vi "RDG822 User(before_screen_branch).vi"() -> ()   [LabVIEW 2021]
panel:
  in  "RemoveReq?":bool
  in  "userID":string="0001"
  out "error out":errorcluster
  in  "E:\\Study\\НИР_Маг\\FP":path=path "E:/Study/НИР_Маг/FP"
  in  "error in":errorcluster
  in  "PhaseDBL":dbl format="%.3f"
  in  "OK":bool
  out "Screen\nPhase":picture
  out "PhaseStr":string="5.0000"
  in  "LowL":dbl=-2.5 format="%.4f"
  in  "Offset":dbl format="%.4f"
  out "Screen\nOffset-LowL":picture
  out "Offset-LowL":string="5.0000"
  in  "Offset/LowL":bool
  in  "HighL":dbl=1.0 format="%.4f"
  in  "Ampl":dbl=5.0 format="%.4f"
  out "Screen\nAmpl-HighL":picture
  out "Ampl-HighL":string="5.0000"
  in  "Ampl/HighL":bool
  in  "Freq":dbl=1.0 format="%.18f"
  in  "Period":dbl=1.0 format="%_8g"
  out "Screen\nFreq/Period":picture
  out "Freq-Period":string="1,000000000"
  in  "Freq/Period":bool
  in  "Left":bool
  in  "Right":bool
  in  "Out2":bool
  in  "Out1":bool
  out "Screen":picture
  in  "Menu":bool
  in  "Home":bool
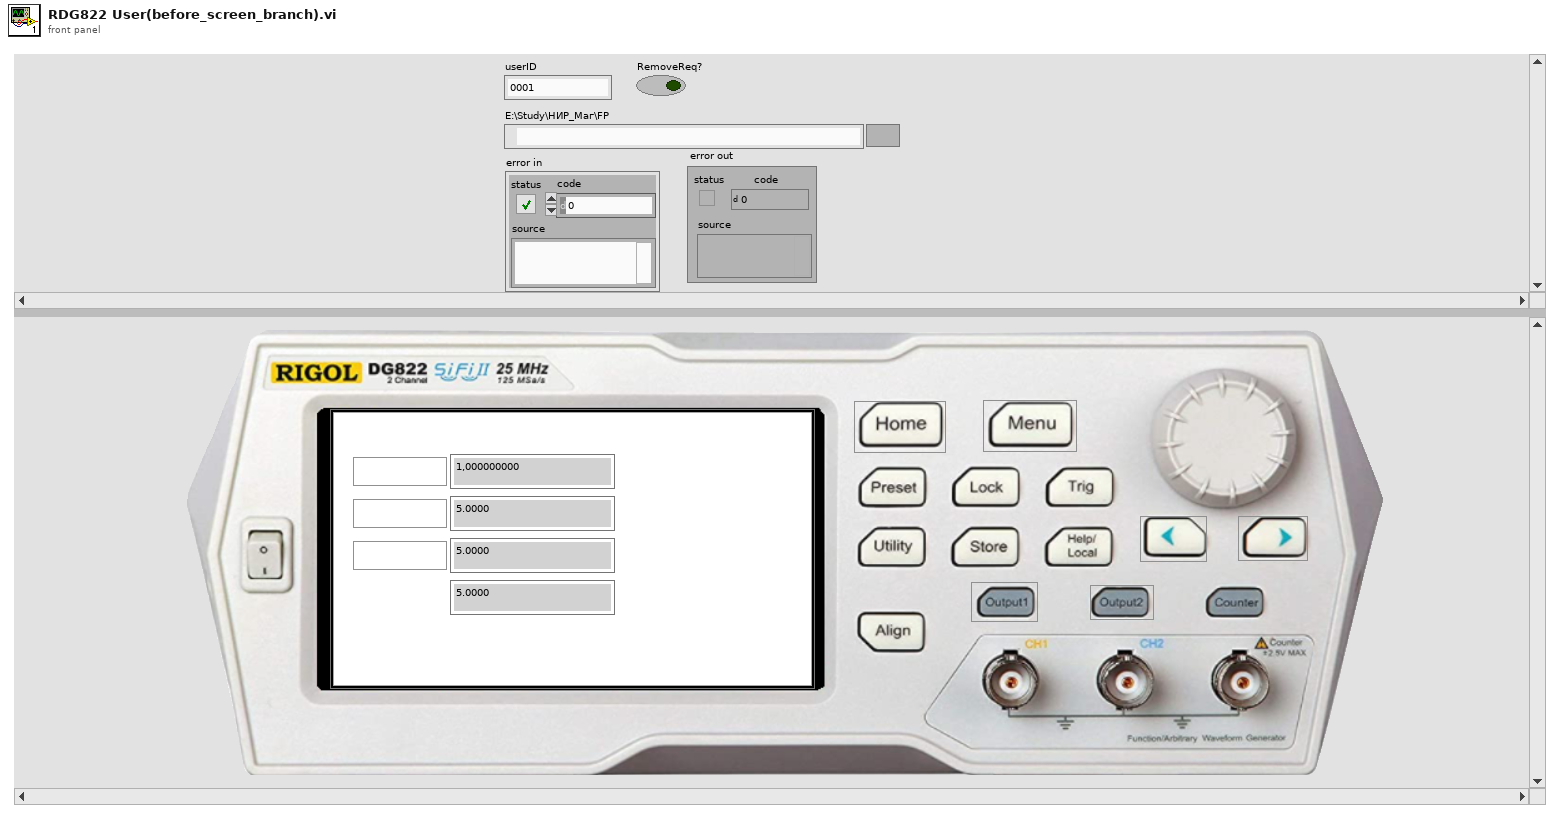
[diagram p1: front panel]
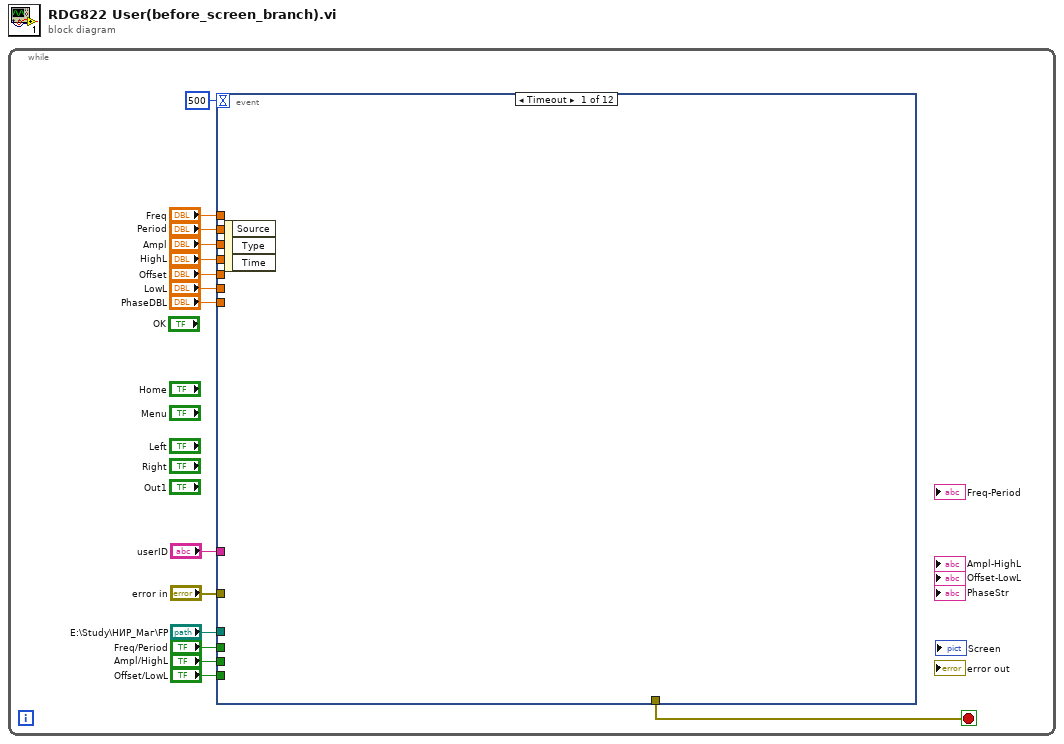
[diagram p0: block diagram]
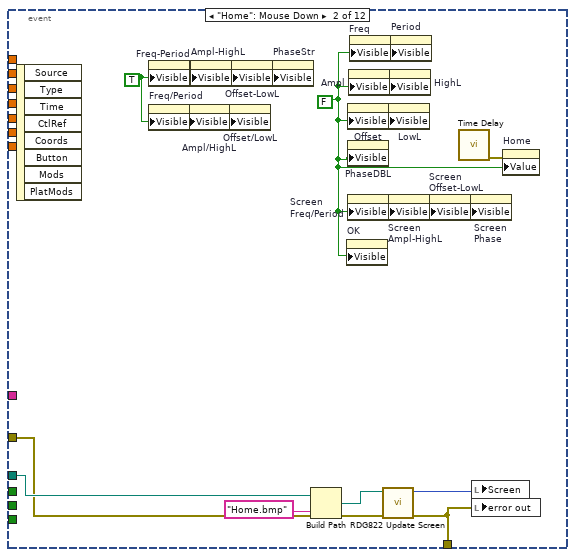
[diagram p2: hidden frame]
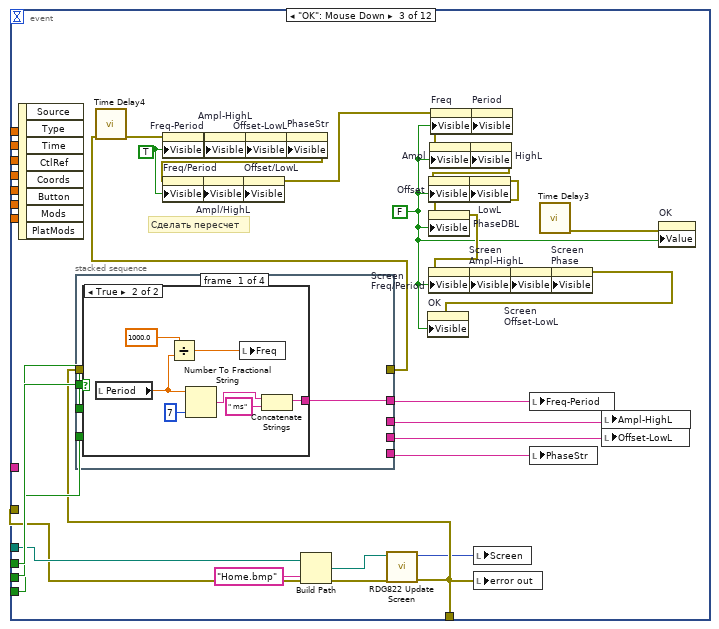
[diagram p3: hidden frame]
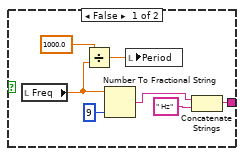
[diagram p4: hidden frame]
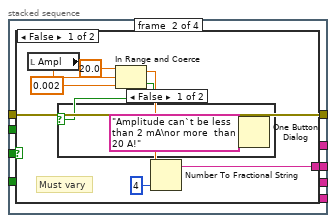
[diagram p5: hidden frame]
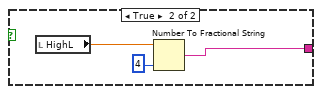
[diagram p7: hidden frame]
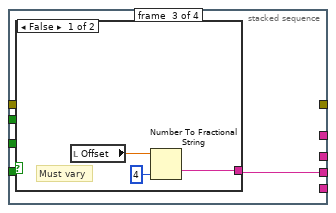
[diagram p8: hidden frame]
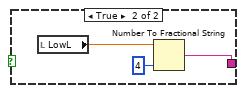
[diagram p9: hidden frame]
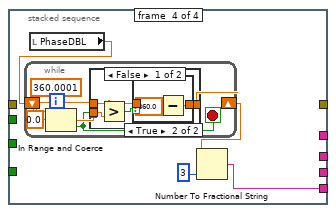
[diagram p10: hidden frame]
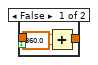
[diagram p11: hidden frame]
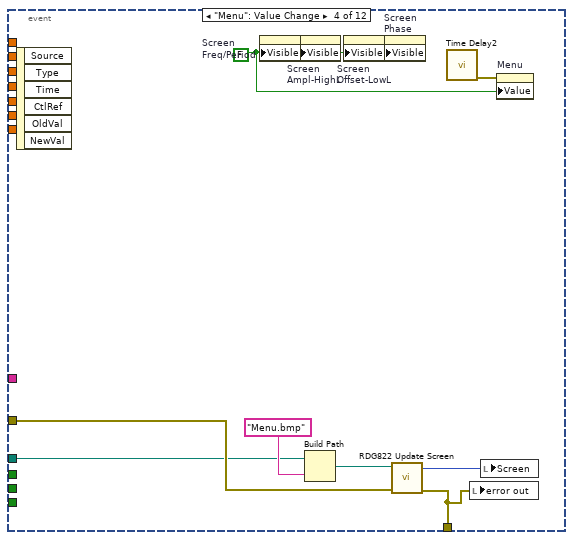
[diagram p13: hidden frame]
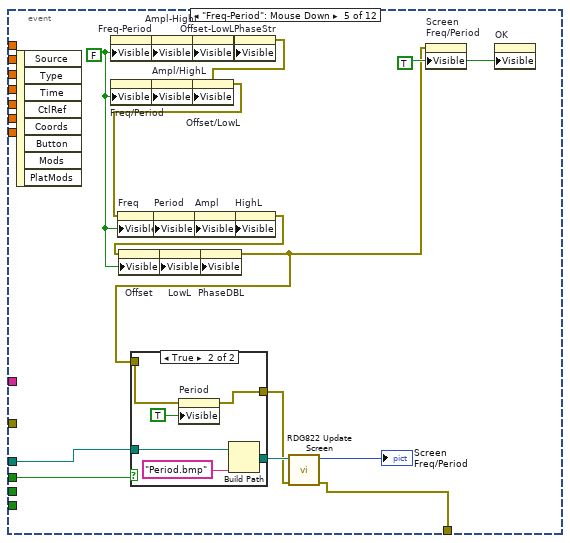
[diagram p14: hidden frame]
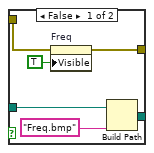
[diagram p15: hidden frame]
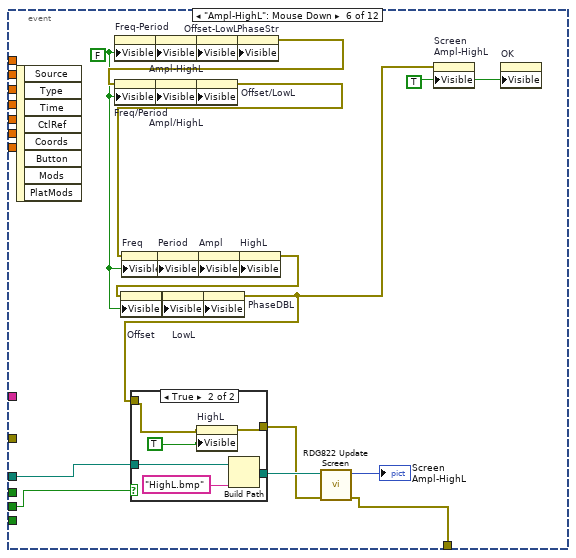
[diagram p16: hidden frame]
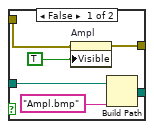
[diagram p17: hidden frame]
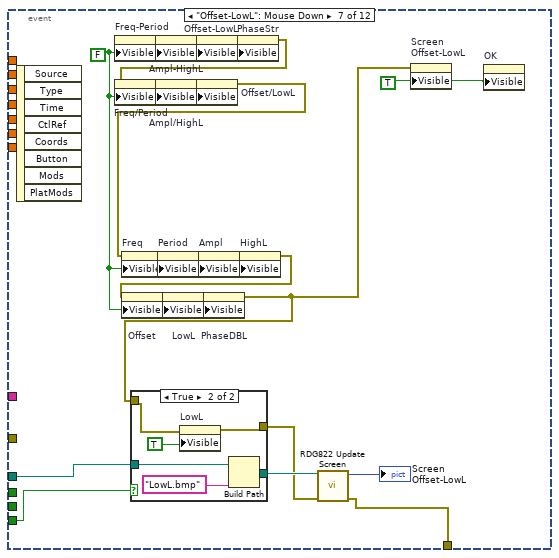
[diagram p18: hidden frame]
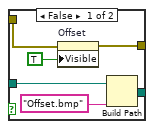
[diagram p19: hidden frame]
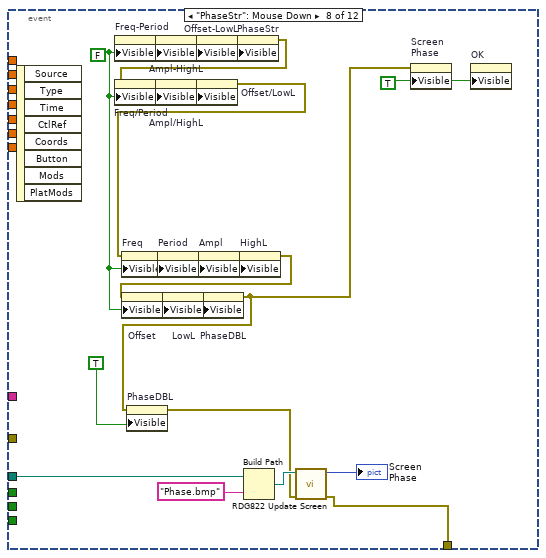
[diagram p20: hidden frame]
diagram:
  n1 = while {
    stop <- w15 stop-if-true
    n2 = event shown="[0] Timeout" {
      selector: _ -> [_ _ _ _ _ _ _ _ _ _ _ _]
      dyn-events: _ -> [_ _ _ _ _ _ _ _ _ _ _ _]
      timeout: 500 -> [_ _ _ _ _ _ _ _ _ _ _ _]
      tunnel: [_ w19 w28 w120 w127 w161 w195 w229 _ _ w296 w374] -> w15
      tunnel: "error in" -> [_ w18 w27 w122 _ _ _ _ _ _ w306 _]
      tunnel: "E:\\Study\\НИР_Маг\\FP" -> [_ w20 w29 w121 w148 w182 w216 w238 _ _ w288 w373]
      tunnel: "Freq/Period" -> [_ _ w35 _ w146 _ _ _ _ _ w325 _]
      tunnel: "Ampl/HighL" -> [_ _ w34 _ _ w177 _ _ _ _ w326 _]
      tunnel: "Freq" -> [_ _ _ _ _ _ _ _ _ _ w324 _]
      tunnel: "Ampl" -> [_ _ _ _ _ _ _ _ _ _ w322 _]
      tunnel: "Period" -> [_ _ _ _ _ _ _ _ _ _ w323 _]
      tunnel: "HighL" -> [_ _ _ _ _ _ _ _ _ _ w318 _]
      tunnel: "Offset/LowL" -> [_ _ w33 _ _ _ w203 _ _ _ w321 _]
      tunnel: "Offset" -> [_ _ _ _ _ _ _ _ _ _ w320 _]
      tunnel: "LowL" -> [_ _ _ _ _ _ _ _ _ _ w319 _]
      tunnel: "PhaseDBL" -> [_ _ _ _ _ _ _ _ _ _ w312 _]
      tunnel: "userID" -> [_ _ _ _ _ _ _ _ _ _ w301 _]
      event Timeout {
        n3 = event-data() -> ()  [unwired: 1 in, 3 out]
      }
      event "Home": Mouse Down {
        w23 = TRUE ("Visible")
        w22 = FALSE ("Visible")
        n4 = event-data() -> ()  [unwired: 1 in, 8 out]
        n5 = property on="Freq-Period" class="Str"("Visible"=w23) -> ()  [unwired: 2 in, 2 out]
        n6 = property on="Freq/Period" class="Bool (strict)"("Visible"=w23) -> ()  [unwired: 2 in, 2 out]
        n7 = property on="Ampl/HighL" class="Bool (strict)"("Visible"=w23) -> ()  [unwired: 2 in, 2 out]
        n8 = property on="Ampl-HighL" class="Str"("Visible"=w23) -> ()  [unwired: 2 in, 2 out]
        n9 = property on="Offset/LowL" class="Bool (strict)"("Visible"=w23) -> ()  [unwired: 2 in, 2 out]
        n10 = property on="Offset-LowL" class="Str"("Visible"=w23) -> ()  [unwired: 2 in, 2 out]
        n11 = property on="PhaseStr" class="Str"("Visible"=w23) -> ()  [unwired: 2 in, 2 out]
        n12 = Build Path(base path=w20, name or relative path="Home.bmp") -> (appended path=w17:path)
        n13 = property on="OK" class="Bool (strict)"("Visible"=w22) -> ()  [unwired: 2 in, 2 out]
        n14 = property on="Offset" class="DigNum (strict)"("Visible"=w22) -> ()  [unwired: 2 in, 2 out]
        n15 = property on="PhaseDBL" class="DigNum (strict)"("Visible"=w22) -> ()  [unwired: 2 in, 2 out]
        n16 = property on="Screen\nFreq/Period" class="Pict"("Visible"=w22) -> ()  [unwired: 2 in, 2 out]
        n17 = property on="Ampl" class="DigNum (strict)"("Visible"=w22) -> ()  [unwired: 2 in, 2 out]
        n18 = property on="Freq" class="DigNum (strict)"("Visible"=w22) -> ()  [unwired: 2 in, 2 out]
        n19 = call "RDG822 Update Screen.vi"("error in"=w18, "Path to file"=w17) -> ("error out"=w19:errorcluster, "Screen"=w16:picture)  [unwired: 8 in]
        n20 = property on="LowL" class="DigNum (strict)"("Visible"=w22) -> ()  [unwired: 2 in, 2 out]
        n21 = property on="Screen\nAmpl-HighL" class="Pict"("Visible"=w22) -> ()  [unwired: 2 in, 2 out]
        n22 = property on="HighL" class="DigNum (strict)"("Visible"=w22) -> ()  [unwired: 2 in, 2 out]
        n23 = property on="Period" class="DigNum (strict)"("Visible"=w22) -> ()  [unwired: 2 in, 2 out]
        n24 = property on="Screen\nOffset-LowL" class="Pict"("Visible"=w22) -> ()  [unwired: 2 in, 2 out]
        n25 = call "Time Delay"() -> ("error out"=w24:errorcluster)  [unwired: 11 in]
        n26 = property on="Screen\nPhase" class="Pict"("Visible"=w22) -> ()  [unwired: 2 in, 2 out]
        n27 = local write "Screen"(w16) -> ()
        n28 = local write "error out"(w19) -> ()
        n29 = property on="Home" class="Bool (strict)"(error in=w24, "Value"=w22) -> ()  [unwired: 1 in, 2 out]
      }
      event "OK": Mouse Down {
        w59 = TRUE ("Visible")
        w39 = FALSE ("Visible")
        # "Сделать пересчет"
        n30 = event-data() -> ()  [unwired: 1 in, 8 out]
        n31 = Build Path(base path=w29, name or relative path="Home.bmp") -> (appended path=w26:path)
        n32 = call "RDG822 Update Screen.vi"("error in"=w27, "Path to file"=w26) -> ("error out"=w28:errorcluster, "Screen"=w25:picture)  [unwired: 8 in]
        n33 = stacked-sequence {
          tunnel: [_ _ w92 _] -> w38
          tunnel: [_ w79 _ _] -> w37
          tunnel: [w62 _ _ _] -> w36
          tunnel: w35 -> [w61 _ _ _]
          tunnel: w34 -> [_ w78 _ _]
          tunnel: w33 -> [_ _ w91 _]
          tunnel: [_ w77 _ _] -> w32
          tunnel: w28 -> [_ w77 _ _]
          tunnel: [_ _ _ w101] -> w31
          frame #0 {
            n34 = case shown="True" w61 {
              tunnel: [w64 w71] -> w62
              frame False {
                n35 = local read "Freq"() -> (w67:dbl)
                n36 = Divide(x=1000.0, y=w67) -> (x/y=w66:dbl)
                n37 = Number To Fractional String(number=w67, precision (6)=i16 9) -> (F-format string=w63:string)  [unwired: 2 in]
                n38 = local write "Period"(w66) -> ()
                n39 = Concatenate Strings(w63, " Hz" ("string")) -> (w64:string)
              }
              frame True {
                n40 = local read "Period"() -> (w74:dbl)
                n41 = Divide(x=1000.0, y=w74) -> (x/y=w73:dbl)
                n42 = Number To Fractional String(number=w74, precision (6)=i16 7) -> (F-format string=w70:string)  [unwired: 2 in]
                n43 = local write "Freq"(w73) -> ()
                n44 = Concatenate Strings(w70, " ms" ("string")) -> (w71:string)
              }
            }
          }
          frame #1 {
            n45 = case shown="False" w78 {
              tunnel: [w85 w88] -> w79
              frame False {
                # "Must vary"
                n46 = local read "Ampl"() -> (w84:dbl)
                n47 = In Range and Coerce(upper limit=20.0, x=w84, lower limit=0.002 ("t")) -> (coerced(x)=w81:dbl, In Range?=w80:bool)
                n48 = case shown="False" w80 {
                  frame False {
                    n49 = One Button Dialog(message="Amplitude can`t be less than 2 mA\nor more  than 20 A!") -> ()  [unwired: 1 in, 1 out]
                  }
                  frame True {
                  }
                }
                n50 = Number To Fractional String(number=w81, precision (6)=i16 4) -> (F-format string=w85:string)  [unwired: 2 in]
              }
              frame True {
                n51 = local read "HighL"() -> (w89:dbl)
                n52 = Number To Fractional String(number=w89, precision (6)=i16 4) -> (F-format string=w88:string)  [unwired: 2 in]
              }
            }
          }
          frame #2 {
            n53 = case shown="False" w91 {
              tunnel: [w94 w98] -> w92
              frame False {
                # "Must vary"
                n54 = local read "Offset"() -> (w95:dbl)
                n55 = Number To Fractional String(number=w95, precision (6)=i16 4) -> (F-format string=w94:string)  [unwired: 2 in]
              }
              frame True {
                n56 = local read "LowL"() -> (w96:dbl)
                n57 = Number To Fractional String(number=w96, precision (6)=i16 4) -> (F-format string=w98:string)  [unwired: 2 in]
              }
            }
          }
          frame #3 {
            n58 = local read "PhaseDBL"() -> (w100:dbl)
            n59 = while {
              shift-right: [w103] -> w99
              shift-left: w100 -> [w105]
              stop <- w104 stop-if-true
              w106 = 360.0001 ("upper limit")
              n60 = In Range and Coerce(upper limit=w106, x=w105, lower limit=0.0) -> (In Range?=w104:bool)  [unwired: 1 out]
              n61 = case shown="False" w104 {
                tunnel: w106 -> [w111 _]
                tunnel: w105 -> [w109 w118]
                tunnel: [w108 w118] -> w103
                frame False {
                  n62 = Greater?(x=w109, y=w111) -> (0:w110:bool)
                  n63 = case shown="True" w110 {
                    tunnel: w109 -> [w113 w115]
                    tunnel: [w112 w116] -> w108
                    frame False {
                      n64 = Add(x=w113, y=360.0) -> (x+y=w112:dbl)
                    }
                    frame True {
                      n65 = Subtract(x=w115, y=360.0) -> (x-y=w116:dbl)
                    }
                  }
                }
                frame True {
                }
              }
            }
            n66 = Number To Fractional String(number=w99, precision (6)=i16 3) -> (F-format string=w101:string)  [unwired: 2 in]
          }
        }
        n67 = call "Time Delay4"("error in (no error)"=w32) -> ("error out"=w58:errorcluster)  [unwired: 10 in]
        n68 = property on="Freq-Period" class="Str"(error in=w58, "Visible"=w59) -> (error out=w57:errorcluster)  [unwired: 1 in, 1 out]
        n69 = property on="Ampl-HighL" class="Str"(error in=w57, "Visible"=w59) -> (error out=w56:errorcluster)  [unwired: 1 in, 1 out]
        n70 = property on="Offset-LowL" class="Str"(error in=w56, "Visible"=w59) -> (error out=w55:errorcluster)  [unwired: 1 in, 1 out]
        n71 = property on="PhaseStr" class="Str"(error in=w55, "Visible"=w59) -> (error out=w54:errorcluster)  [unwired: 1 in, 1 out]
        n72 = property on="Freq/Period" class="Bool (strict)"(error in=w54, "Visible"=w59) -> (error out=w53:errorcluster)  [unwired: 1 in, 1 out]
        n73 = property on="Ampl/HighL" class="Bool (strict)"(error in=w53, "Visible"=w59) -> (error out=w52:errorcluster)  [unwired: 1 in, 1 out]
        n74 = property on="Offset/LowL" class="Bool (strict)"(error in=w52, "Visible"=w59) -> (error out=w51:errorcluster)  [unwired: 1 in, 1 out]
        n75 = property on="Freq" class="DigNum (strict)"(error in=w51, "Visible"=w39) -> (error out=w50:errorcluster)  [unwired: 1 in, 1 out]
        n76 = property on="Period" class="DigNum (strict)"(error in=w50, "Visible"=w39) -> (error out=w49:errorcluster)  [unwired: 1 in, 1 out]
        n77 = property on="Ampl" class="DigNum (strict)"(error in=w49, "Visible"=w39) -> (error out=w48:errorcluster)  [unwired: 1 in, 1 out]
        n78 = property on="HighL" class="DigNum (strict)"(error in=w48, "Visible"=w39) -> (error out=w47:errorcluster)  [unwired: 1 in, 1 out]
        n79 = property on="Offset" class="DigNum (strict)"(error in=w47, "Visible"=w39) -> (error out=w46:errorcluster)  [unwired: 1 in, 1 out]
        n80 = property on="LowL" class="DigNum (strict)"(error in=w46, "Visible"=w39) -> (error out=w41:errorcluster)  [unwired: 1 in, 1 out]
        n81 = property on="PhaseDBL" class="DigNum (strict)"(error in=w41, "Visible"=w39) -> (error out=w40:errorcluster)  [unwired: 1 in, 1 out]
        n82 = property on="Screen\nFreq/Period" class="Pict"(error in=w40, "Visible"=w39) -> (error out=w45:errorcluster)  [unwired: 1 in, 1 out]
        n83 = property on="Screen\nAmpl-HighL" class="Pict"(error in=w45, "Visible"=w39) -> (error out=w44:errorcluster)  [unwired: 1 in, 1 out]
        n84 = local write "Screen"(w25) -> ()
        n85 = local write "error out"(w28) -> ()
        n86 = property on="Screen\nOffset-LowL" class="Pict"(error in=w44, "Visible"=w39) -> (error out=w43:errorcluster)  [unwired: 1 in, 1 out]
        n87 = local write "Freq-Period"(w36) -> ()
        n88 = local write "PhaseStr"(w31) -> ()
        n89 = call "Time Delay3"() -> ("error out"=w60:errorcluster)  [unwired: 11 in]
        n90 = property on="Screen\nPhase" class="Pict"(error in=w43, "Visible"=w39) -> (error out=w42:errorcluster)  [unwired: 1 in, 1 out]
        n91 = property on="OK" class="Bool (strict)"(error in=w42, "Visible"=w39) -> ()  [unwired: 1 in, 2 out]
        n92 = local write "Ampl-HighL"(w37) -> ()
        n93 = local write "Offset-LowL"(w38) -> ()
        n94 = property on="OK" class="Bool (strict)"(error in=w60, "Value"=w39) -> ()  [unwired: 1 in, 2 out]
      }
      event "Menu": Value Change {
        w125 = FALSE ("Visible")
        n95 = event-data() -> ()  [unwired: 1 in, 6 out]
        n96 = property on="Screen\nFreq/Period" class="Pict"("Visible"=w125) -> ()  [unwired: 2 in, 2 out]
        n97 = property on="Screen\nAmpl-HighL" class="Pict"("Visible"=w125) -> ()  [unwired: 2 in, 2 out]
        n98 = Build Path(base path=w121, name or relative path="Menu.bmp") -> (appended path=w123:path)
        n99 = property on="Screen\nOffset-LowL" class="Pict"("Visible"=w125) -> ()  [unwired: 2 in, 2 out]
        n100 = property on="Screen\nPhase" class="Pict"("Visible"=w125) -> ()  [unwired: 2 in, 2 out]
        n101 = call "RDG822 Update Screen.vi"("error in"=w122, "Path to file"=w123) -> ("error out"=w120:errorcluster, "Screen"=w119:picture)  [unwired: 8 in]
        n102 = call "Time Delay2"() -> ("error out"=w126:errorcluster)  [unwired: 11 in]
        n103 = local write "error out"(w120) -> ()
        n104 = local write "Screen"(w119) -> ()
        n105 = property on="Menu" class="Bool (strict)"(error in=w126, "Value"=w125) -> ()  [unwired: 1 in, 2 out]
      }
      event "Freq-Period": Mouse Down {
        w134 = TRUE ("Visible")
        w132 = FALSE ("Visible")
        n106 = event-data() -> ()  [unwired: 1 in, 8 out]
        n107 = property on="Freq-Period" class="Str"("Visible"=w132) -> (error out=w145:errorcluster)  [unwired: 2 in, 1 out]
        n108 = property on="Ampl-HighL" class="Str"(error in=w145, "Visible"=w132) -> (error out=w141:errorcluster)  [unwired: 1 in, 1 out]
        n109 = property on="Offset-LowL" class="Str"(error in=w141, "Visible"=w132) -> (error out=w136:errorcluster)  [unwired: 1 in, 1 out]
        n110 = property on="PhaseStr" class="Str"(error in=w136, "Visible"=w132) -> (error out=w135:errorcluster)  [unwired: 1 in, 1 out]
        n111 = property on="Freq/Period" class="Bool (strict)"(error in=w135, "Visible"=w132) -> (error out=w144:errorcluster)  [unwired: 1 in, 1 out]
        n112 = property on="Ampl/HighL" class="Bool (strict)"(error in=w144, "Visible"=w132) -> (error out=w140:errorcluster)  [unwired: 1 in, 1 out]
        n113 = property on="Offset/LowL" class="Bool (strict)"(error in=w140, "Visible"=w132) -> (error out=w139:errorcluster)  [unwired: 1 in, 1 out]
        n114 = property on="Freq" class="DigNum (strict)"(error in=w139, "Visible"=w132) -> (error out=w147:errorcluster)  [unwired: 1 in, 1 out]
        n115 = property on="Period" class="DigNum (strict)"(error in=w147, "Visible"=w132) -> (error out=w143:errorcluster)  [unwired: 1 in, 1 out]
        n116 = property on="Ampl" class="DigNum (strict)"(error in=w143, "Visible"=w132) -> (error out=w142:errorcluster)  [unwired: 1 in, 1 out]
        n117 = property on="HighL" class="DigNum (strict)"(error in=w142, "Visible"=w132) -> (error out=w138:errorcluster)  [unwired: 1 in, 1 out]
        n118 = property on="Offset" class="DigNum (strict)"(error in=w138, "Visible"=w132) -> (error out=w137:errorcluster)  [unwired: 1 in, 1 out]
        n119 = property on="LowL" class="DigNum (strict)"(error in=w137, "Visible"=w132) -> (error out=w133:errorcluster)  [unwired: 1 in, 1 out]
        n120 = property on="PhaseDBL" class="DigNum (strict)"(error in=w133, "Visible"=w132) -> (error out=w131:errorcluster)  [unwired: 1 in, 1 out]
        n121 = case shown="True" w146 {
          tunnel: [w154 w160] -> w129
          tunnel: w148 -> [w152 w158]
          tunnel: w131 -> [w150 w156]
          tunnel: [w149 w155] -> w128
          frame False {
            n122 = property on="Freq" class="DigNum (strict)"(error in=w150, "Visible"=TRUE) -> (error out=w149:errorcluster)  [unwired: 1 in, 1 out]
            n123 = Build Path(base path=w152, name or relative path="Freq.bmp") -> (appended path=w154:path)
          }
          frame True {
            n124 = property on="Period" class="DigNum (strict)"(error in=w156, "Visible"=TRUE) -> (error out=w155:errorcluster)  [unwired: 1 in, 1 out]
            n125 = Build Path(base path=w158, name or relative path="Period.bmp") -> (appended path=w160:path)
          }
        }
        n126 = call "RDG822 Update Screen.vi"("error in"=w128, "Path to file"=w129) -> ("error out"=w127:errorcluster, "Screen"=→"Screen\nFreq/Period":picture)  [unwired: 8 in]
        n127 = property on="Screen\nFreq/Period" class="Pict"(error in=w131, "Visible"=w134) -> ()  [unwired: 1 in, 2 out]
        n128 = property on="OK" class="Bool (strict)"("Visible"=w134) -> ()  [unwired: 2 in, 2 out]
      }
      event "Ampl-HighL": Mouse Down {
        w166 = FALSE ("Visible")
        w168 = TRUE ("Visible")
        n129 = event-data() -> ()  [unwired: 1 in, 8 out]
        n130 = property on="Freq-Period" class="Str"("Visible"=w166) -> (error out=w180:errorcluster)  [unwired: 2 in, 1 out]
        n131 = property on="Ampl-HighL" class="Str"(error in=w180, "Visible"=w166) -> (error out=w175:errorcluster)  [unwired: 1 in, 1 out]
        n132 = property on="Offset-LowL" class="Str"(error in=w175, "Visible"=w166) -> (error out=w170:errorcluster)  [unwired: 1 in, 1 out]
        n133 = property on="PhaseStr" class="Str"(error in=w170, "Visible"=w166) -> (error out=w169:errorcluster)  [unwired: 1 in, 1 out]
        n134 = property on="Freq/Period" class="Bool (strict)"(error in=w169, "Visible"=w166) -> (error out=w179:errorcluster)  [unwired: 1 in, 1 out]
        n135 = property on="Ampl/HighL" class="Bool (strict)"(error in=w179, "Visible"=w166) -> (error out=w174:errorcluster)  [unwired: 1 in, 1 out]
        n136 = property on="Offset/LowL" class="Bool (strict)"(error in=w174, "Visible"=w166) -> (error out=w173:errorcluster)  [unwired: 1 in, 1 out]
        n137 = property on="Freq" class="DigNum (strict)"(error in=w173, "Visible"=w166) -> (error out=w181:errorcluster)  [unwired: 1 in, 1 out]
        n138 = property on="Period" class="DigNum (strict)"(error in=w181, "Visible"=w166) -> (error out=w178:errorcluster)  [unwired: 1 in, 1 out]
        n139 = property on="Ampl" class="DigNum (strict)"(error in=w178, "Visible"=w166) -> (error out=w176:errorcluster)  [unwired: 1 in, 1 out]
        n140 = property on="HighL" class="DigNum (strict)"(error in=w176, "Visible"=w166) -> (error out=w172:errorcluster)  [unwired: 1 in, 1 out]
        n141 = property on="Offset" class="DigNum (strict)"(error in=w172, "Visible"=w166) -> (error out=w171:errorcluster)  [unwired: 1 in, 1 out]
        n142 = property on="LowL" class="DigNum (strict)"(error in=w171, "Visible"=w166) -> (error out=w167:errorcluster)  [unwired: 1 in, 1 out]
        n143 = property on="PhaseDBL" class="DigNum (strict)"(error in=w167, "Visible"=w166) -> (error out=w165:errorcluster)  [unwired: 1 in, 1 out]
        n144 = case shown="True" w177 {
          tunnel: [w188 w194] -> w163
          tunnel: w182 -> [w186 w192]
          tunnel: w165 -> [w184 w191]
          tunnel: [w183 w189] -> w162
          frame False {
            n145 = property on="Ampl" class="DigNum (strict)"(error in=w184, "Visible"=TRUE) -> (error out=w183:errorcluster)  [unwired: 1 in, 1 out]
            n146 = Build Path(base path=w186, name or relative path="Ampl.bmp") -> (appended path=w188:path)
          }
          frame True {
            n147 = property on="HighL" class="DigNum (strict)"(error in=w191, "Visible"=TRUE) -> (error out=w189:errorcluster)  [unwired: 1 in, 1 out]
            n148 = Build Path(base path=w192, name or relative path="HighL.bmp") -> (appended path=w194:path)
          }
        }
        n149 = call "RDG822 Update Screen.vi"("error in"=w162, "Path to file"=w163) -> ("error out"=w161:errorcluster, "Screen"=→"Screen\nAmpl-HighL":picture)  [unwired: 8 in]
        n150 = property on="Screen\nAmpl-HighL" class="Pict"(error in=w165, "Visible"=w168) -> ()  [unwired: 1 in, 2 out]
        n151 = property on="OK" class="Bool (strict)"("Visible"=w168) -> ()  [unwired: 2 in, 2 out]
      }
      event "Offset-LowL": Mouse Down {
        w200 = FALSE ("Visible")
        w202 = TRUE ("Visible")
        n152 = event-data() -> ()  [unwired: 1 in, 8 out]
        n153 = property on="Freq-Period" class="Str"("Visible"=w200) -> (error out=w214:errorcluster)  [unwired: 2 in, 1 out]
        n154 = property on="Ampl-HighL" class="Str"(error in=w214, "Visible"=w200) -> (error out=w210:errorcluster)  [unwired: 1 in, 1 out]
        n155 = property on="Offset-LowL" class="Str"(error in=w210, "Visible"=w200) -> (error out=w205:errorcluster)  [unwired: 1 in, 1 out]
        n156 = property on="PhaseStr" class="Str"(error in=w205, "Visible"=w200) -> (error out=w204:errorcluster)  [unwired: 1 in, 1 out]
        n157 = property on="Freq/Period" class="Bool (strict)"(error in=w204, "Visible"=w200) -> (error out=w213:errorcluster)  [unwired: 1 in, 1 out]
        n158 = property on="Ampl/HighL" class="Bool (strict)"(error in=w213, "Visible"=w200) -> (error out=w209:errorcluster)  [unwired: 1 in, 1 out]
        n159 = property on="Offset/LowL" class="Bool (strict)"(error in=w209, "Visible"=w200) -> (error out=w208:errorcluster)  [unwired: 1 in, 1 out]
        n160 = property on="Freq" class="DigNum (strict)"(error in=w208, "Visible"=w200) -> (error out=w215:errorcluster)  [unwired: 1 in, 1 out]
        n161 = property on="Period" class="DigNum (strict)"(error in=w215, "Visible"=w200) -> (error out=w212:errorcluster)  [unwired: 1 in, 1 out]
        n162 = property on="Ampl" class="DigNum (strict)"(error in=w212, "Visible"=w200) -> (error out=w211:errorcluster)  [unwired: 1 in, 1 out]
        n163 = property on="HighL" class="DigNum (strict)"(error in=w211, "Visible"=w200) -> (error out=w206:errorcluster)  [unwired: 1 in, 1 out]
        n164 = property on="Offset" class="DigNum (strict)"(error in=w206, "Visible"=w200) -> (error out=w207:errorcluster)  [unwired: 1 in, 1 out]
        n165 = property on="LowL" class="DigNum (strict)"(error in=w207, "Visible"=w200) -> (error out=w201:errorcluster)  [unwired: 1 in, 1 out]
        n166 = property on="PhaseDBL" class="DigNum (strict)"(error in=w201, "Visible"=w200) -> (error out=w199:errorcluster)  [unwired: 1 in, 1 out]
        n167 = case shown="True" w203 {
          tunnel: [w222 w228] -> w197
          tunnel: w216 -> [w220 w226]
          tunnel: w199 -> [w218 w225]
          tunnel: [w217 w223] -> w196
          frame False {
            n168 = property on="Offset" class="DigNum (strict)"(error in=w218, "Visible"=TRUE) -> (error out=w217:errorcluster)  [unwired: 1 in, 1 out]
            n169 = Build Path(base path=w220, name or relative path="Offset.bmp") -> (appended path=w222:path)
          }
          frame True {
            n170 = property on="LowL" class="DigNum (strict)"(error in=w225, "Visible"=TRUE) -> (error out=w223:errorcluster)  [unwired: 1 in, 1 out]
            n171 = Build Path(base path=w226, name or relative path="LowL.bmp") -> (appended path=w228:path)
          }
        }
        n172 = call "RDG822 Update Screen.vi"("error in"=w196, "Path to file"=w197) -> ("error out"=w195:errorcluster, "Screen"=→"Screen\nOffset-LowL":picture)  [unwired: 8 in]
        n173 = property on="Screen\nOffset-LowL" class="Pict"(error in=w199, "Visible"=w202) -> ()  [unwired: 1 in, 2 out]
        n174 = property on="OK" class="Bool (strict)"("Visible"=w202) -> ()  [unwired: 2 in, 2 out]
      }
      event "PhaseStr": Mouse Down {
        w235 = FALSE ("Visible")
        w237 = TRUE ("Visible")
        n175 = event-data() -> ()  [unwired: 1 in, 8 out]
        n176 = property on="Freq-Period" class="Str"("Visible"=w235) -> (error out=w250:errorcluster)  [unwired: 2 in, 1 out]
        n177 = property on="Ampl-HighL" class="Str"(error in=w250, "Visible"=w235) -> (error out=w246:errorcluster)  [unwired: 1 in, 1 out]
        n178 = property on="Offset-LowL" class="Str"(error in=w246, "Visible"=w235) -> (error out=w241:errorcluster)  [unwired: 1 in, 1 out]
        n179 = property on="PhaseStr" class="Str"(error in=w241, "Visible"=w235) -> (error out=w240:errorcluster)  [unwired: 1 in, 1 out]
        n180 = property on="Freq/Period" class="Bool (strict)"(error in=w240, "Visible"=w235) -> (error out=w249:errorcluster)  [unwired: 1 in, 1 out]
        n181 = property on="Ampl/HighL" class="Bool (strict)"(error in=w249, "Visible"=w235) -> (error out=w245:errorcluster)  [unwired: 1 in, 1 out]
        n182 = property on="Offset/LowL" class="Bool (strict)"(error in=w245, "Visible"=w235) -> (error out=w244:errorcluster)  [unwired: 1 in, 1 out]
        n183 = property on="Freq" class="DigNum (strict)"(error in=w244, "Visible"=w235) -> (error out=w251:errorcluster)  [unwired: 1 in, 1 out]
        n184 = property on="Period" class="DigNum (strict)"(error in=w251, "Visible"=w235) -> (error out=w248:errorcluster)  [unwired: 1 in, 1 out]
        n185 = property on="Ampl" class="DigNum (strict)"(error in=w248, "Visible"=w235) -> (error out=w247:errorcluster)  [unwired: 1 in, 1 out]
        n186 = property on="HighL" class="DigNum (strict)"(error in=w247, "Visible"=w235) -> (error out=w242:errorcluster)  [unwired: 1 in, 1 out]
        n187 = property on="Offset" class="DigNum (strict)"(error in=w242, "Visible"=w235) -> (error out=w243:errorcluster)  [unwired: 1 in, 1 out]
        n188 = property on="LowL" class="DigNum (strict)"(error in=w243, "Visible"=w235) -> (error out=w236:errorcluster)  [unwired: 1 in, 1 out]
        n189 = property on="PhaseDBL" class="DigNum (strict)"(error in=w236, "Visible"=w235) -> (error out=w234:errorcluster)  [unwired: 1 in, 1 out]
        n190 = property on="PhaseDBL" class="DigNum (strict)"(error in=w234, "Visible"=TRUE) -> (error out=w230:errorcluster)  [unwired: 1 in, 1 out]
        n191 = Build Path(base path=w238, name or relative path="Phase.bmp") -> (appended path=w232:path)
        n192 = call "RDG822 Update Screen.vi"("error in"=w230, "Path to file"=w232) -> ("error out"=w229:errorcluster, "Screen"=→"Screen\nPhase":picture)  [unwired: 8 in]
        n193 = property on="Screen\nPhase" class="Pict"(error in=w234, "Visible"=w237) -> ()  [unwired: 1 in, 2 out]
        n194 = property on="OK" class="Bool (strict)"("Visible"=w237) -> ()  [unwired: 2 in, 2 out]
      }
      event "Freq/Period": Value Change {
        n195 = event-data() -> ("NewVal"=w252:bool)  [unwired: 1 in, 5 out]
        n196 = case shown="False" w252 {
          tunnel: [w256 w262] -> w253
          frame False {
            # "Must vary"
            n197 = local read "Period"() -> (w259:dbl)
            n198 = Divide(x=1000.0, y=w259) -> (x/y=w257:dbl)
            n199 = Number To Fractional String(number=w257, precision (6)=i16 9) -> (F-format string=w254:string)  [unwired: 2 in]
            n200 = local write "Freq"(w257) -> ()
            n201 = Concatenate Strings(w254, " Hz" ("string")) -> (w256:string)
          }
          frame True {
            # "Must vary"
            n202 = local read "Freq"() -> (w265:dbl)
            n203 = Divide(x=1000.0, y=w265) -> (x/y=w264:dbl)
            n204 = local write "Period"(w264) -> ()
            n205 = Number To Fractional String(number=w264, precision (6)=i16 7) -> (F-format string=w261:string)  [unwired: 2 in]
            n206 = Concatenate Strings(w261, " ms" ("string")) -> (w262:string)
          }
        }
        n207 = local write "Freq-Period"(w253) -> ()
      }
      event "Ampl/HighL", "Offset/LowL": Value Change {
        # "Сделать пересчет"
        n208 = event-data() -> ("NewVal"=w270:bool)  [unwired: 1 in, 5 out]
        n209 = case shown="False" w270 {
          tunnel: [w274 w278] -> w271
          frame False {
            # "Must vary"
            n210 = local read "Offset"() -> (w275:dbl)
            n211 = Number To Fractional String(number=w275, precision (6)=i16 4) -> (F-format string=w274:string)  [unwired: 2 in]
          }
          frame True {
            n212 = local read "LowL"() -> (w276:dbl)
            n213 = Number To Fractional String(number=w276, precision (6)=i16 4) -> (F-format string=w278:string)  [unwired: 2 in]
          }
        }
        n214 = case shown="False" w270 {
          tunnel: [w280 w284] -> w272
          frame False {
            # "Must vary"
            n215 = local read "Ampl"() -> (w281:dbl)
            n216 = Number To Fractional String(number=w281, precision (6)=i16 4) -> (F-format string=w280:string)  [unwired: 2 in]
          }
          frame True {
            n217 = local read "HighL"() -> (w282:dbl)
            n218 = Number To Fractional String(number=w282, precision (6)=i16 4) -> (F-format string=w284:string)  [unwired: 2 in]
          }
        }
        n219 = local read "Ampl/HighL"() -> (w269:bool)
        n220 = local read "Offset/LowL"() -> (w268:bool)
        n221 = local write "Ampl-HighL"(w272) -> ()
        n222 = local write "Offset-LowL"(w271) -> ()
        n223 = local write "Offset/LowL"(w269) -> ()
        n224 = local write "Ampl/HighL"(w268) -> ()
      }
      event "Out1": Mouse Down {
        w294 = u16 2 items=["Send", "Read", "Download", "Remove"] ("Send/Read/Download/Remove")
        w295 = u16 0 items=["Send", "Read", "Download", "Remove"] ("Send/Read/Download/Remove")
        w309 = FALSE ("Visible")
        w300 = 1 items=["Channel 1"=1, "Channel 2"=2] ("Output Channel (1: Channel 1)")
        # "Placeholder"
        n225 = event-data() -> ()  [unwired: 1 in, 8 out]
        n226 = case shown="True" w325 {
          tunnel: w324 -> [w368 _]
          tunnel: w323 -> [_ w370]
          tunnel: [w368 w369] -> w302
          frame False {
          }
          frame True {
            n227 = Divide(x=1000.0, y=w370) -> (x/y=w369:dbl)
          }
        }
        n228 = case shown="True" w326 {
          tunnel: w322 -> [w354 _]
          tunnel: w318 -> [_ w366]
          tunnel: [w355 w360] -> w303
          tunnel: w319 -> [_ w365]
          frame False {
            n229 = In Range and Coerce(upper limit=20.0, x=w354, lower limit=0.002 ("t")) -> (coerced(x)=w355:dbl, In Range?=w356:bool)
            n230 = case shown="False" w356 {
              frame False {
                n231 = One Button Dialog(message="Amplitude can`t be less than 2 mA\nor more than 20 A!") -> ()  [unwired: 1 in, 1 out]
              }
              frame True {
              }
            }
          }
          frame True {
            n232 = Subtract(x=w366, y=w365) -> (x-y=w362:dbl)
            n233 = In Range and Coerce(upper limit=20.0, x=w362, lower limit=0.002 ("t")) -> (coerced(x)=w360:dbl, In Range?=w361:bool)
            n234 = case shown="False" w361 {
              frame False {
                n235 = One Button Dialog(message="Amplitude can`t be less than 2 mA\nor greater than 20 A!") -> ()  [unwired: 1 in, 1 out]
              }
              frame True {
              }
            }
          }
        }
        n236 = case shown="True" w321 {
          tunnel: w320 -> [w348 _]
          tunnel: w319 -> [_ w353]
          tunnel: [w348 w349] -> w304
          tunnel: w318 -> [_ w350]
          frame False {
          }
          frame True {
            n237 = Add(x=w350, y=w353) -> (x+y=w352:dbl)
            n238 = Divide(x=w352, y=2.0) -> (x/y=w349:dbl)
          }
        }
        n239 = while {
          shift-right: [w332] -> w305
          shift-left: w312 -> [w334]
          stop <- w333 stop-if-true
          w335 = 360.0001 ("upper limit")
          n240 = In Range and Coerce(upper limit=w335, x=w334, lower limit=0.0) -> (In Range?=w333:bool)  [unwired: 1 out]
          n241 = case shown="True" w333 {
            tunnel: w335 -> [w340 _]
            tunnel: w334 -> [w338 w347]
            tunnel: [w337 w347] -> w332
            frame False {
              n242 = Greater?(x=w338, y=w340) -> (0:w339:bool)
              n243 = case shown="True" w339 {
                tunnel: w338 -> [w342 w344]
                tunnel: [w341 w345] -> w337
                frame False {
                  n244 = Add(x=w342, y=360.0) -> (x+y=w341:dbl)
                }
                frame True {
                  n245 = Subtract(x=w344, y=360.0) -> (x-y=w345:dbl)
                }
              }
            }
            frame True {
            }
          }
        }
        n246 = call "PlaceholderForSin.vi"("Phase (0 Degree)"=w305, "Output Channel (1: Channel 1)"=w300, "Offset (0)"=w304, "error in (no error)"=w306, "Amplitude (5 Vpp)"=w303, "Frequency (1000 Hz)"=w302) -> ("error out"=w299:errorcluster, "resulting string"=w298:string)  [unwired: 4 in]
        n247 = call "HTTPGetRequest_Inst.vi"("Send/Read/Download/Remove"=w295, "error in (no error)"=w299, "userdata="=w298, "userID"=w301) -> ("error out"=w287:errorcluster, "ReqNum"=w285:string)  [unwired: 5 in, 1 out]
        n248 = Build Path(base path=w288, name or relative path=path "Results") -> (appended path=w290:path)
        n249 = call "QueryDoneFlag.vi"("error in (no error)"=w287, "ReqNum"=w285) -> ("error out"=w286:errorcluster)  [unwired: 9 in]
        n250 = call "HTTPGetRequest_Inst.vi"("Send/Read/Download/Remove"=w294, "Path to FP"=w290, "error in (no error)"=w286, "ReqNum"=w285) -> ("error out"=w307:errorcluster)  [unwired: 5 in, 2 out]
        n251 = call "UnZipFile.vi"("error in (no error)"=w307, "Zip name"=w285, "Path to FP"=w290) -> ("error out"=w297:errorcluster, "File path"=w292:path)  [unwired: 7 in]
        n252 = case shown="True" "RemoveReq?" {
          tunnel: w297 -> [w327 w331]
          tunnel: [w327 w330] -> w296
          tunnel: w285 -> [_ w328]
          frame False {
          }
          frame True {
            w329 = u16 3 items=["Send", "Read", "Download", "Remove"] ("Send/Read/Download/Remove")
            n253 = call "HTTPGetRequest_Inst.vi"("Send/Read/Download/Remove"=w329, "error in (no error)"=w331, "ReqNum"=w328) -> ("error out"=w330:errorcluster)  [unwired: 6 in, 2 out]
          }
        }
        n254 = property on="Freq-Period" class="Str"(error in=w296, "Visible"=w309) -> (error out=w315:errorcluster)  [unwired: 1 in, 1 out]
        n255 = property on="Freq/Period" class="Bool (strict)"(error in=w296, "Visible"=w309) -> (error out=w311:errorcluster)  [unwired: 1 in, 1 out]
        n256 = property on="Ampl-HighL" class="Str"(error in=w315, "Visible"=w309) -> (error out=w314:errorcluster)  [unwired: 1 in, 1 out]
        n257 = call "Time Delay5"() -> ("error out"=w317:errorcluster)  [unwired: 11 in]
        n258 = property on="Ampl/HighL" class="Bool (strict)"(error in=w311, "Visible"=w309) -> (error out=w310:errorcluster)  [unwired: 1 in, 1 out]
        n259 = call "RDG822 Update Screen.vi"("error in"=w296, "Path to file"=w292) -> ("error out"=w308:errorcluster, "Screen"=w293:picture)  [unwired: 8 in]
        n260 = property on="Offset-LowL" class="Str"(error in=w314, "Visible"=w309) -> (error out=w313:errorcluster)  [unwired: 1 in, 1 out]
        n261 = local write "error out"(w308) -> ()
        n262 = property on="Offset/LowL" class="Bool (strict)"(error in=w310, "Visible"=w309) -> ()  [unwired: 1 in, 2 out]
        n263 = property on="Out1" class="Bool (strict)"(error in=w317, "Value"=FALSE ("Out1")) -> ()  [unwired: 1 in, 2 out]
        n264 = local write "Screen"(w293) -> ()
        n265 = property on="PhaseStr" class="Str"(error in=w313, "Visible"=w309) -> ()  [unwired: 1 in, 2 out]
      }
      event "Out2": Value Change {
        (unwired) 2 items=["Channel 1"=1, "Channel 2"=2] ("Output Channel (1: Channel 1)")
        # "Same as Out1 eventually"
        n266 = event-data() -> ()  [unwired: 1 in, 6 out]
        n267 = call "Time Delay"() -> ("error out"=w372:errorcluster)  [unwired: 11 in]
        n268 = call "RDG822 Update Screen(Old).vi"("Path"=w373, "error in"=w372) -> ("error out"=w374:errorcluster, "Screen"=w375:picture)  [unwired: 8 in]
        n269 = local write "error out"(w374) -> ()
        n270 = local write "Screen"(w375) -> ()
      }
    }
  }
